vi "MSEditor_Script_EnableSearchTool.vi"(7 "Func":enum16{"Init", "GetNext", "Clear"}(ring), 8 "error in (no error)":errorcluster, 11 "search param refnum":T1) -> (0 "error out":errorcluster, 2 "first search":bool)   [LabVIEW 2018]
uses:
  <vilib>/Utility/miscctls.llb/LVPositionTypeDef.ctl
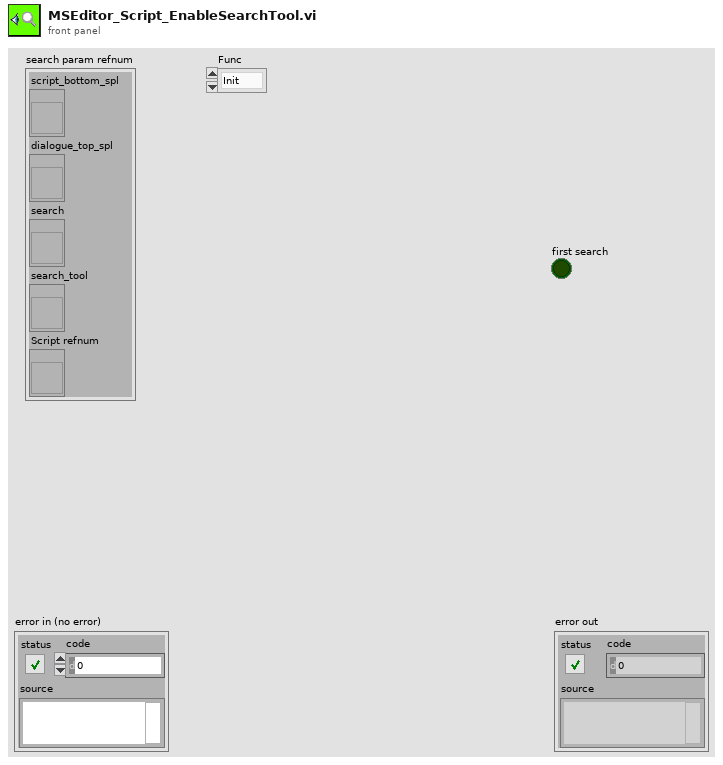
[diagram p1: front panel]
types:
  T1 = cluster{"script_bottom_spl":refnum<vi>, "dialogue_top_spl":refnum<vi>, "search":refnum<vi>, "search_tool":refnum<vi>, "Script refnum":refnum<vi>}
  T2 = typedef "LVPositionTypeDef.ctl" = cluster{"Left":i32, "Top":i32}
  T3 = typedef "LVSelectionTypeDef.ctl" = cluster{"Selection Start":u32, "Selection End":u32}
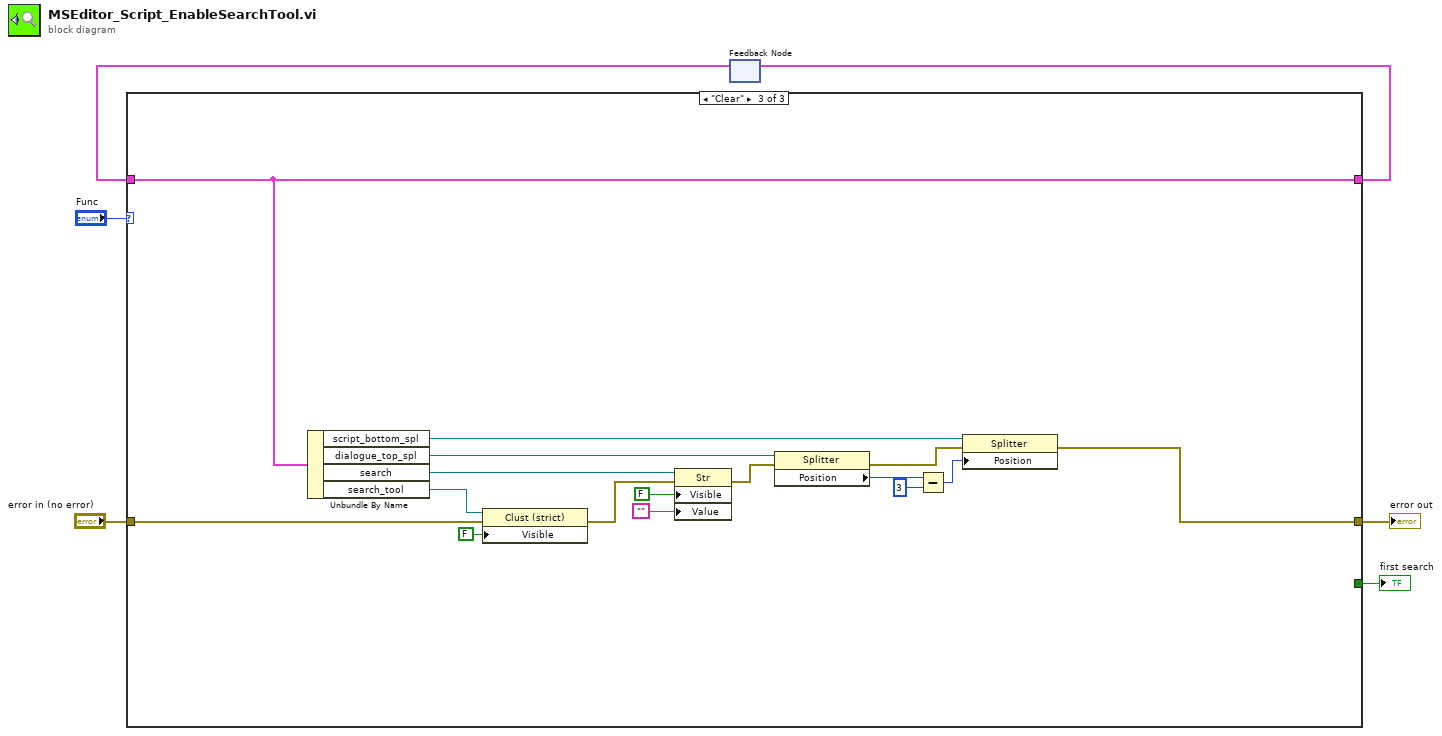
[diagram p0: block diagram]
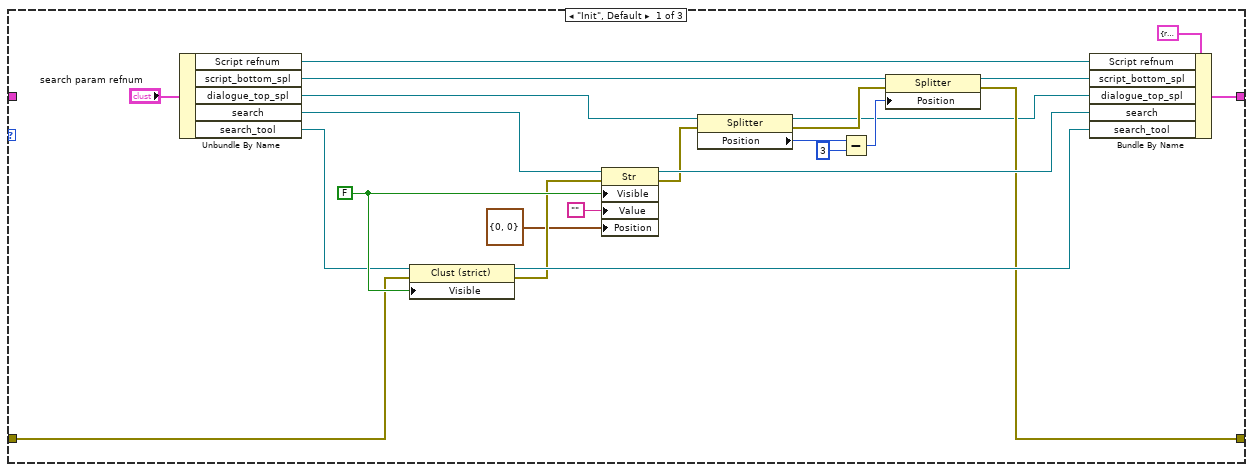
[diagram p2: hidden frame]
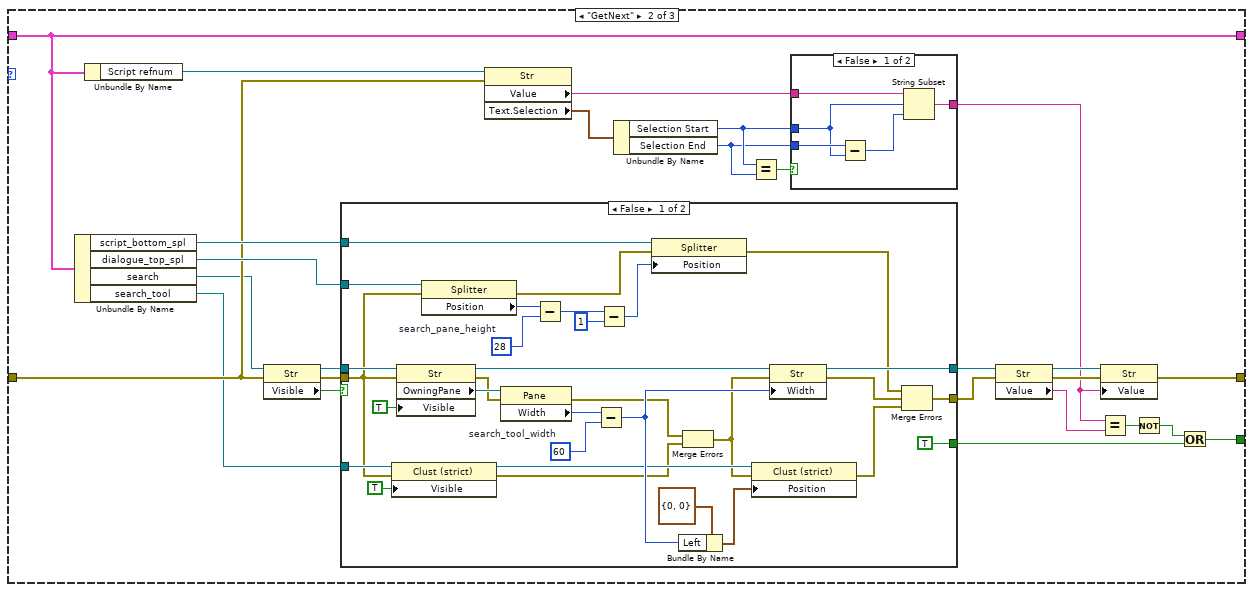
[diagram p3: hidden frame]
diagram:
  n1 = feedback #1() -> (w4:T1)  [unwired: 1 in]
  n2 = case shown="\"Clear\"" "Func" {
    tunnel: [w28 w35 w109] -> w5
    tunnel: w4 -> [_ w35 w109]
    tunnel: [_ w38 _] -> w3
    tunnel: [w18 w37 w95] -> w2
    tunnel: "error in (no error)" -> [w23 w32 w101]
    frame "Init", Default {
      w24 = FALSE ("Visible")
      n3 = Unbundle By Name("search param refnum") -> ("Script refnum"=w8:refnum<vi>, "script_bottom_spl"=w9:refnum<vi>, "dialogue_top_spl"=w10:refnum<vi>, "search"=w11:refnum<vi>, "search_tool"=w12:refnum<vi>)
      n4 = property class="Clust (strict)"(reference=w12, error in=w23, "Visible"=w24) -> (reference out=w20:refnum<vi>, error out=w17:errorcluster)
      n5 = property class="Str"(reference=w11, error in=w17, "Visible"=w24, "Value"="", "Position"=T2 {"Left"=0, "Top"=0}) -> (reference out=w21:refnum<vi>, error out=w15:errorcluster)
      n6 = property class="Splitter"(reference=w10, error in=w15) -> (reference out=w16:refnum<vi>, error out=w19:errorcluster, "Position"=w27:i32)
      n7 = Subtract(x=w27, y=3) -> (x-y=w25:i32)
      n8 = property class="Splitter"(reference=w9, error in=w19, "Position"=w25) -> (reference out=w22:refnum<vi>, error out=w18:errorcluster)
      n9 = Bundle By Name(cluster=T1 {"script_bottom_spl"=refnum, "dialogue_top_spl"=refnum, "search"=refnum, "search_tool"=refnum, "Script refnum"=refnum}, "Script refnum"=w8, "script_bottom_spl"=w22, "dialogue_top_spl"=w16, "search"=w21, "search_tool"=w20) -> (w28:T1)
    }
    frame "GetNext" {
      n10 = Unbundle By Name(w35) -> ("script_bottom_spl"=w34:refnum<vi>, "dialogue_top_spl"=w33:refnum<vi>, "search"=w31:refnum<vi>, "search_tool"=w30:refnum<vi>)
      n11 = Unbundle By Name(w35) -> ("Script refnum"=w36:refnum<vi>)
      n12 = property class="Str"(reference=w31, error in=w32) -> (reference out=w50:refnum<vi>, error out=w48:errorcluster, "Visible"=w49:bool)
      n13 = case shown="False" w49 {
        tunnel: w33 -> [w86 _]
        tunnel: w34 -> [w81 _]
        tunnel: w50 -> [w79 w88]
        tunnel: [w71 w88] -> w47
        tunnel: w48 -> [w59 w87]
        tunnel: [w65 w87] -> w46
        tunnel: [TRUE _] -> w40
        tunnel: w30 -> [w62 _]
        frame False {
          w75 = u32 60  # search_tool_width
          w80 = 28  # search_pane_height
          n14 = property class="Clust (strict)"(reference=w62, error in=w59, "Visible"=TRUE) -> (reference out=w60:refnum<vi>, error out=w57:errorcluster)
          n15 = property class="Str"(reference=w79, error in=w59, "Visible"=TRUE) -> (reference out=w77:refnum<vi>, error out=w69:errorcluster, "OwningPane"=w78:refnum<vi>)
          n16 = property class="Splitter"(reference=w86, error in=w59) -> (error out=w70:errorcluster, "Position"=w83:i32)  [unwired: 1 out]
          n17 = property class="Pane"(reference=w78, error in=w69) -> (error out=w58:errorcluster, "Width"=w76:u32)  [unwired: 1 out]
          n18 = Subtract(x=w83, y=w80) -> (x-y=w85:i32)
          n19 = Subtract(x=w76, y=w75) -> (x-y=w73:u32)
          n20 = Subtract(x=w85, y=u32 1) -> (x-y=w82:u32)
          n21 = property class="Splitter"(reference=w81, error in=w70, "Position"=w82) -> (error out=w67:errorcluster)  [unwired: 1 out]
          n22 = Bundle By Name(cluster=T2 {"Left"=0, "Top"=0} ("Position"), "Left"=w73) -> (w72:T2)
          n23 = Merge Errors(w58, w57) -> (w56:errorcluster)
          n24 = property class="Clust (strict)"(reference=w60, error in=w56, "Position"=w72) -> (error out=w66:errorcluster)  [unwired: 1 out]
          n25 = property class="Str"(reference=w77, error in=w56, "Width"=w73) -> (reference out=w71:refnum<vi>, error out=w68:errorcluster)
          n26 = Merge Errors(w67, w68, w66) -> (w65:errorcluster)
        }
        frame True {
        }
      }
      n27 = property class="Str"(reference=w36, error in=w32) -> ("Value"=w54:string, "Text.Selection"=w55:T3)  [unwired: 2 out]
      n28 = Unbundle By Name(w55) -> ("Selection Start"=w53:u32, "Selection End"=w52:u32)
      n29 = Equal?(x=w53, y=w52) -> (x = y?=w51:bool)
      n30 = case shown="False" w51 {
        tunnel: w54 -> [w93 _]
        tunnel: [w92 _] -> w39
        tunnel: w53 -> [w90 _]
        tunnel: w52 -> [w91 _]
        frame False {
          n31 = Subtract(x=w91, y=w90) -> (x-y=w89:u32)
          n32 = String Subset(string=w93, offset (0)=w90, length (rest)=w89) -> (substring=w92:string)
        }
        frame True {
        }
      }
      n33 = property class="Str"(reference=w47, error in=w46) -> (reference out=w45:refnum<vi>, error out=w44:errorcluster, "Value"=w41:string)
      n34 = Equal?(x=w39, y=w41) -> (x = y?=w43:bool)
      n35 = property class="Str"(reference=w45, error in=w44, "Value"=w39) -> (error out=w37:errorcluster)  [unwired: 1 out]
      n36 = Not(x=w43) -> (.not. x?=w42:bool)
      n37 = Or(x=w42, y=w40) -> (x .or. y?=w38:bool)
    }
    frame "Clear" {
      n38 = Unbundle By Name(w109) -> ("script_bottom_spl"=w105:refnum<vi>, "dialogue_top_spl"=w104:refnum<vi>, "search"=w103:refnum<vi>, "search_tool"=w102:refnum<vi>)
      n39 = property class="Clust (strict)"(reference=w102, error in=w101, "Visible"=FALSE) -> (error out=w100:errorcluster)  [unwired: 1 out]
      n40 = property class="Str"(reference=w103, error in=w100, "Visible"=FALSE, "Value"="") -> (error out=w99:errorcluster)  [unwired: 1 out]
      n41 = property class="Splitter"(reference=w104, error in=w99) -> (error out=w98:errorcluster, "Position"=w108:i32)  [unwired: 1 out]
      n42 = Subtract(x=w108, y=3) -> (x-y=w106:i32)
      n43 = property class="Splitter"(reference=w105, error in=w98, "Position"=w106) -> (error out=w95:errorcluster)  [unwired: 1 out]
    }
  }
  "error out" <- w2
  "first search" <- w3
  n44 = feedback-in #1(w5) -> ()
